vi "LuaVIEW Get Function Documentation.vi"(0 "function path":path, 11 "error in (no error)":errorcluster) -> (4 "documentation":string, 8 "reentrant?":bool, 10 "synopsis":string, 15 "error out":errorcluster)   [LabVIEW 2012]
doc: "Returns the documentation, reentrancy, and synopsis of LuaVIEW function VI given a path to that VI. For this to work, the function must have been documented with the provided editor."
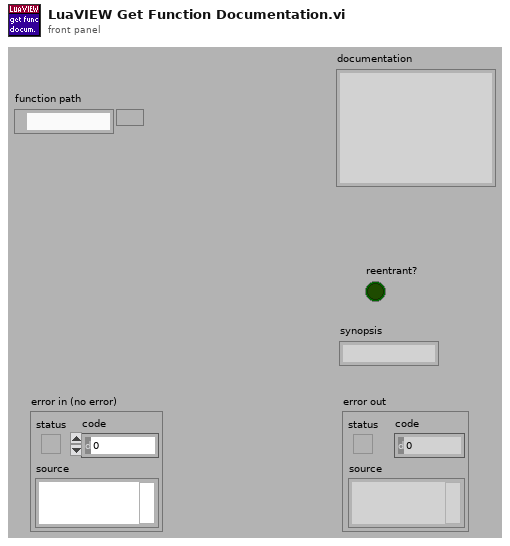
[diagram p1: front panel]
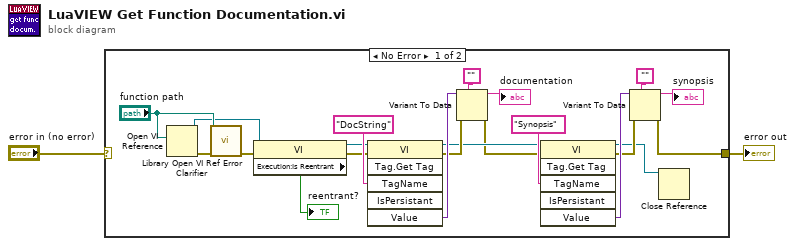
[diagram p0: block diagram]
diagram:
  n1 = case shown="No Error" "error in (no error)" {
    selector: "error in (no error)" -> [_ w24]
    tunnel: [w23 w24] -> w2
    frame No Error {
      n2 = Open VI Reference(vi path="function path") -> (vi reference=w19:refnum<vi>, error out=w22:errorcluster)  [unwired: 5 in]
      n3 = call "Library Open VI Ref Error Clarifier.vi"("VI path"="function path", "called VI error (no error)"=w22) -> ("error out"=w20:errorcluster)  [unwired: 13 in]
      n4 = property class="VI"(reference=w19, error in=w20) -> (reference out=w12:refnum<vi>, error out=w13:errorcluster, "Execution:Is Reentrant"=→"reentrant?":bool)
      n5 = invoke class="VI" method="Tag.Get Tag"(reference=w12, error in=w13, "TagName"="DocString") -> (reference out=w4:refnum<vi>, error out=w15:errorcluster, "Value"=w16:variant)  [unwired: 3 in, 3 out]
      n6 = Variant To Data(error in=w15, type="", Variant=w16) -> (data=→"documentation":string, error out=w3:errorcluster)
      n7 = invoke class="VI" method="Tag.Get Tag"(reference=w4, error in=w3, "TagName"="Synopsis") -> (reference out=w8:refnum<vi>, error out=w9:errorcluster, "Value"=w10:variant)  [unwired: 3 in, 3 out]
      n8 = Variant To Data(error in=w9, type="", Variant=w10) -> (data=→"synopsis":string, error out=w23:errorcluster)
      n9 = Close Reference(reference=w8) -> ()  [unwired: 1 in, 1 out]
    }
    frame Error {
    }
  }
  "error out" <- w2
